vi "Agilent SNA Wait for Operation Complete (OPC).vi"(7 "Agilent SNA & SWP":T1, 8 "error in (no error)":errorcluster, 9 "Timeout, ms (10000)":u32=10000, 11 "VISA Resource Names":T2) -> (0 "error out":errorcluster, 3 "dup VISA Resource Names":T2)   [LabVIEW 2011]
uses:
  TypeDefs/Agilent SNA VISA.ctl
  TypeDefs/Agilent SNA Instrument Info.ctl
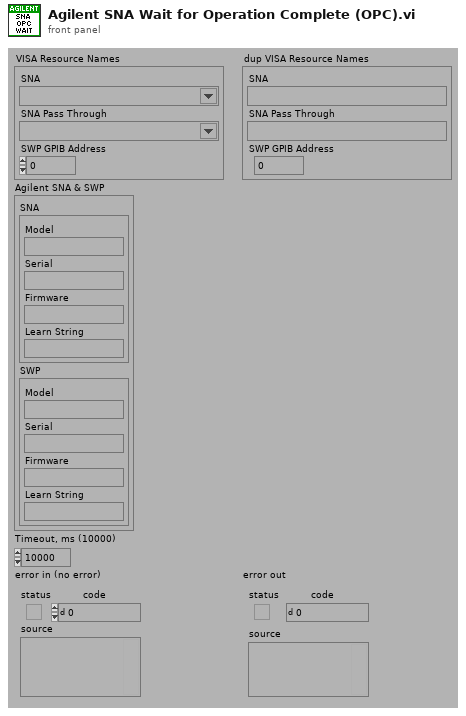
[diagram p1: front panel]
types:
  T1 = typedef "Agilent SNA Instrument Info.ctl" = cluster{"SNA":cluster{"Model":string, "Serial":string, "Firmware":string, "Learn String":string}, "SWP":cluster{"Model":string, "Serial":string, "Firmware":string, "Learn String":string}}
  T2 = typedef "Agilent SNA VISA.ctl" = cluster{"SNA":refnum<visa-resource-name>, "SNA Pass Through":refnum<visa-resource-name>, "SWP GPIB Address":i32}
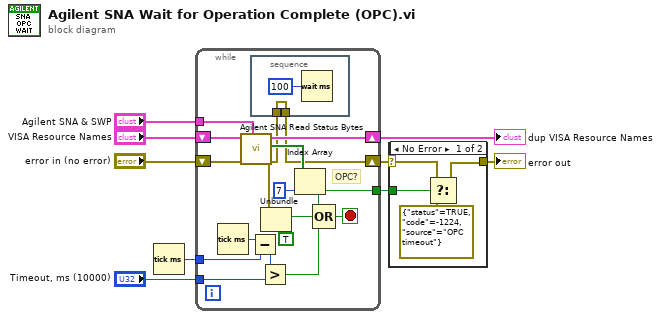
[diagram p0: block diagram]
diagram:
  n1 = Tick Count (ms)() -> (millisecond timer value=w9:u32)
  n2 = while {
    tunnel: [w12] -> w6
    tunnel: "Timeout, ms (10000)" -> [w22]
    tunnel: w9 -> [w25]
    shift-right: [w10] -> w5
    shift-left: "error in (no error)" -> [w19]
    shift-right: [w15] -> w2
    shift-left: "VISA Resource Names" -> [w21]
    tunnel: "Agilent SNA & SWP" -> [w14]
    stop <- w16 stop-if-true
    (unwired) TRUE ("value")
    # "OPC?"
    n3 = Tick Count (ms)() -> (millisecond timer value=w24:u32)
    n4 = call "Agilent SNA Read Status Bytes.vi"("Agilent SNA & SWP"=w14, "error in (no error)"=w19, "VISA Resource Names"=w21) -> ("error out"=w11:errorcluster, "Status Byte"=w20:bool[], "dup VISA Resource Names"=w15:T2)  [unwired: 6 out]
    n5 = Subtract(x=w24, y=w25) -> (x-y=w23:u32)
    n6 = stacked-sequence {
      tunnel: w11 -> [w26]
      tunnel: [w26] -> w10
      frame #0 {
        n7 = Wait (ms)(milliseconds to wait=u32 100) -> ()  [unwired: 1 out]
      }
    }
    n8 = Greater?(x=w23, y=w22) -> (0:w17:bool)
    n9 = Unbundle(w11) -> ("status"=w18:bool)  [unwired: 2 out]
    n10 = Index Array(array=w20, index=7) -> (element=w12:bool)
    n11 = Compound Arithmetic op=OR(w12, w18, w17) -> (w16:bool)
  }
  "dup VISA Resource Names" <- w2
  n12 = case shown="No Error" w5 {
    selector: w5 -> [w30 w32]
    tunnel: w6 -> [w31 _]
    tunnel: [w29 w32] -> w4
    frame No Error {
      n13 = Select(t=w30, s=w31, f=errorcluster {"status"=TRUE, "code"=-1224, "source"="OPC timeout"}) -> (s? t:f=w29:errorcluster)
    }
    frame Error {
    }
  }
  "error out" <- w4
